vi "RT Host Interleaving.vi"() -> ()   [LabVIEW 2012]
uses:
  <vilib>/rvi/interface/nirviOpenFPGA/nirviOpenFPGA.xnode
  <vilib>/rvi/interface/nirviCloseFPGA/nirviCloseFPGA.xnode
  <vilib>/rvi/interface/nirviMethod/nirviMethod.xnode
  <vilib>/rvi/interface/nirviReadWriteControl/nirviReadWriteControl.xnode
  FPGA Interleaving.vi
  <vilib>/rvi/errors/niLvFpgaMergeErrorWithErrorCode.vi
  <vilib>/rvi/errors/niLvFpgaAdjustHostInterfaceError.vi
  <vilib>/LabVIEW Targets/FPGA/cRIO/shared/nicrio_ModuleControls/nicrio_cRIO-9234_DataRatesRing2.ctl
  NiFpgaLv.dll
  <vilib>/Utility/error.llb/Error Cluster From Error Code.vi
  <vilib>/FPGAPlugInAG/cRIO-9074/niLvFpga_ReadFifo_cRIO-9074.vi
  <vilib>/FPGAPlugInAG/cRIO-9074/niLvFpga_Reset_cRIO-9074.vi
  <vilib>/FPGAPlugInAG/cRIO-9074/niLvFpga_ConfigureFifo_cRIO-9074.vi
  <vilib>/FPGAPlugInAG/cRIO-9074/niLvFpga_Run_cRIO-9074.vi
  <vilib>/FPGAPlugInAG/cRIO-9074/niLvFpga_Close_cRIO-9074.vi
panel:
  in  "Data Rate":T1=1 items=["51.200 kS/s (NI 9234)"=1, "25.600 kS/s (NI 9234)"=2, "17.067 kS/s (NI 9234)"=3, "12.800 kS/s (NI 9234)"=4, "10.240 kS/s (NI 9234)"=5, "8.533 kS/s (NI 9234)"=6, "7.314 kS/s (NI 9234)"=7, "6.400 kS/s (NI 9234)"=8, "5.689 kS/s (NI 9234)"=9, "5.120 kS/s (NI 9234)"=10, "4.654 kS/s (NI 9234)"=11, "4.267 kS/s (NI 9234)"=12, "3.938 kS/s (NI 9234)"=13, "3.657 kS/s (NI 9234)"=14, "3.413 kS/s (NI 9234)"=15, "3.200 kS/s (NI 9234)"=16, "3.012 kS/s (NI 9234)"=17, "2.845 kS/s (NI 9234)"=18, "2.695 kS/s (NI 9234)"=19, "2.560 kS/s (NI 9234)"=20, "2.438 kS/s (NI 9234)"=21, "2.328 kS/s (NI 9234)"=22, "2.226 kS/s (NI 9234)"=23, "2.133 kS/s (NI 9234)"=24, "2.048 kS/s (NI 9234)"=25, "1.969 kS/s (NI 9234)"=26, "1.896 kS/s (NI 9234)"=27, "1.829 kS/s (NI 9234)"=28, "1.765 kS/s (NI 9234)"=29, "1.707 kS/s (NI 9234)"=30, "1.652 kS/s (NI 9234)"=31]
  out "error out":errorcluster
  out "Overflow Count":u32
  in  "stop":bool
  in  "Samples per Channel":u32=1000
  out "Accelerometer Data":dbl[][](graph)
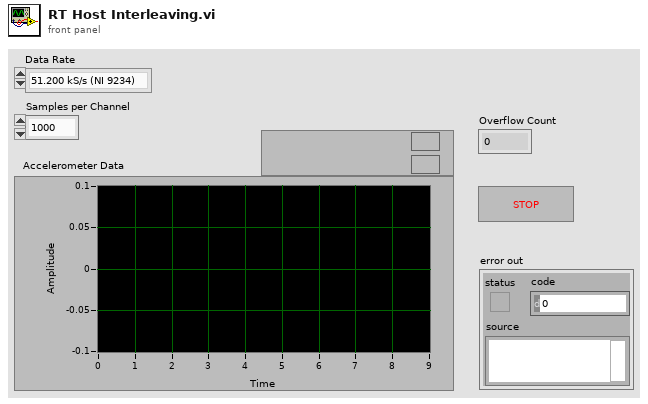
[diagram p1: front panel]
types:
  T1 = typedef "nicrio_cRIO-9234_DataRatesRing2.ctl" = u8
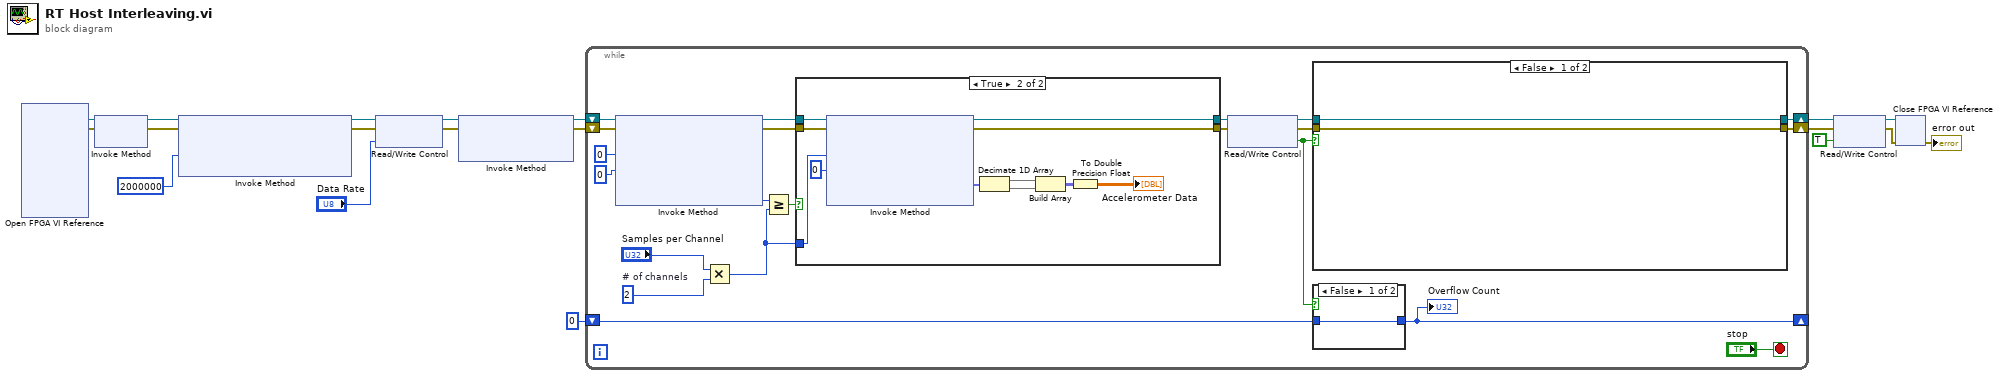
[diagram p0: block diagram]
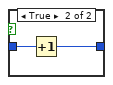
[diagram p2: hidden frame]
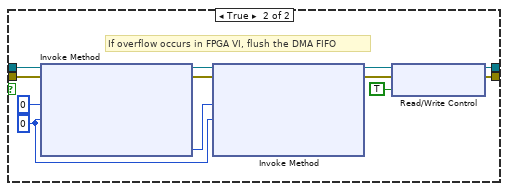
[diagram p4: hidden frame]
diagram:
  n1 = xnode "Open FPGA VI Reference"() -> ("FPGA VI Reference Out"=w2:refnum<k20>, "error out"=w1:errorcluster)  [unwired: 2 in]
  n2 = xnode "Invoke Method"("FPGA VI Reference In"=w2, "error in"=w1) -> ("FPGA VI Reference Out"=w15:refnum<k20>, "error out"=w14:errorcluster)
  n3 = xnode "Invoke Method"("FPGA VI Reference In"=w15, "error in"=w14, "Requested Depth"=u32 2000000 ("Depth")) -> ("FPGA VI Reference Out"=w9:refnum<k20>, "error out"=w8:errorcluster)  [unwired: 1 out]
  n4 = xnode "Read/Write Control"("FPGA VI Reference In"=w9, "error in"=w8, "Data Rate"="Data Rate") -> ("FPGA VI Reference Out"=w19:refnum<k20>, "error out"=w17:errorcluster)
  n5 = xnode "Invoke Method"("FPGA VI Reference In"=w19, "error in"=w17) -> ("FPGA VI Reference Out"=w7:refnum<k20>, "error out"=w18:errorcluster)  [unwired: 1 in]
  n6 = while {
    shift-right: [w35] -> w13
    shift-left: w7 -> [w27]
    shift-right: [w26] -> w6
    shift-left: w18 -> [w38]
    shift-right: [w22] -> _
    shift-left: u32 0 -> [w23]
    stop <- "stop" stop-if-true
    w39 = u32 2  # # of channels
    n7 = xnode "Invoke Method"("FPGA VI Reference In"=w27, "error in"=w38, "Number of Elements"=u32 0, "Timeout (ms)"=0) -> ("FPGA VI Reference Out"=w31:refnum<k20>, "error out"=w30:errorcluster, "Elements Remaining"=w33:u32)  [unwired: 1 out]
    n8 = Multiply(x="Samples per Channel", y=w39) -> (x*y=w20:u32)
    n9 = Greater Or Equal?(x=w33, y=w20) -> (x >= y?=w32:bool)
    n10 = case shown="True" w32 {
      tunnel: w31 -> [w45 w56]
      tunnel: w30 -> [w44 w55]
      tunnel: w20 -> [_ w54]
      tunnel: [w45 w47] -> w29
      tunnel: [w44 w46] -> w28
      frame False {
      }
      frame True {
        n11 = xnode "Invoke Method"("FPGA VI Reference In"=w56, "error in"=w55, "Number of Elements"=w54, "Timeout (ms)"=0) -> ("FPGA VI Reference Out"=w47:refnum<k20>, "error out"=w46:errorcluster, "Data"=w48:fxp<+/-,24,4>[])  [unwired: 1 out]
        n12 = Decimate 1D Array "Decimate 1D Array"(w48) -> (w49:fxp<+/-,24,4>[], w50:fxp<+/-,24,4>[])
        n13 = Build Array "Build Array"(w49, w50) -> (w51:fxp<+/-,24,4>[][])
        n14 = To Double Precision Float(number=w51) -> (double precision float=→"Accelerometer Data":dbl[][])
      }
    }
    n15 = xnode "Read/Write Control"("FPGA VI Reference In"=w29, "error in"=w28) -> ("FPGA VI Reference Out"=w37:refnum<k20>, "error out"=w36:errorcluster, "Overflow?"=w21:bool)
    n16 = case shown="False" w21 {
      tunnel: w37 -> [w58 w70]
      tunnel: w36 -> [w57 w69]
      tunnel: [w58 w65] -> w35
      tunnel: [w57 w64] -> w26
      frame False {
      }
      frame True {
        w61 = 0 ("Timeout (ms)")
        # "If overflow occurs in FPGA VI, flush the DMA FIFO"
        n17 = xnode "Invoke Method"("FPGA VI Reference In"=w70, "error in"=w69, "Number of Elements"=u32 0, "Timeout (ms)"=w61) -> ("FPGA VI Reference Out"=w68:refnum<k20>, "error out"=w67:errorcluster, "Elements Remaining"=w62:u32)  [unwired: 1 out]
        n18 = xnode "Invoke Method"("FPGA VI Reference In"=w68, "error in"=w67, "Number of Elements"=w62, "Timeout (ms)"=w61) -> ("FPGA VI Reference Out"=w60:refnum<k20>, "error out"=w59:errorcluster)  [unwired: 2 out]
        n19 = xnode "Read/Write Control"("FPGA VI Reference In"=w60, "error in"=w59, "DMA Cleared?"=TRUE ("Reset")) -> ("FPGA VI Reference Out"=w65:refnum<k20>, "error out"=w64:errorcluster)
      }
    }
    n20 = case shown="False" w21 {
      tunnel: w23 -> [w41 w43]
      tunnel: [w41 w42] -> w22
      frame False {
      }
      frame True {
        n21 = Increment(x=w43) -> (x+1=w42:u32)
      }
    }
    "Overflow Count" <- w22
  }
  n22 = xnode "Read/Write Control"("FPGA VI Reference In"=w13, "error in"=w6, "stop"=TRUE) -> ("FPGA VI Reference Out"=w12:refnum<k20>, "error out"=w11:errorcluster)
  n23 = xnode "Close FPGA VI Reference"("FPGA VI Reference In"=w12, "error in"=w11) -> ("error out"=→"error out":errorcluster)
